vi "UpdateStatusChannels.vi"(8 "error in (no error)":errorcluster, 9 "success?":bool, 10 "Data":u8[](array[numeric]), 11 "StatusFIFO":refnum<k33>) -> (0 "error out":errorcluster)   [LabVIEW 2015, in "Diagnostics Addon Engine.lvlib"]
uses:
  Diagnostics Addon Engine.lvlib
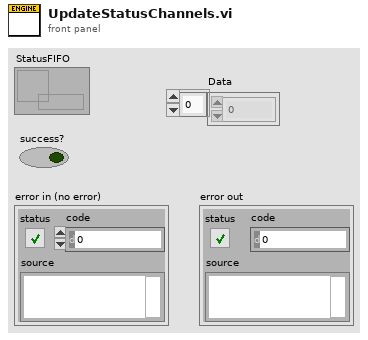
[diagram p1: front panel]
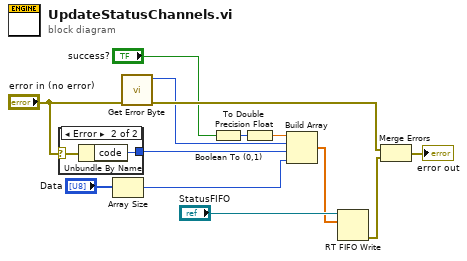
[diagram p0: block diagram]
diagram:
  n1 = case shown="Error" "error in (no error)" {
    selector: "error in (no error)" -> [_ w15]
    tunnel: [_ w14] -> w3
    frame No Error {
    }
    frame Error {
      n2 = Unbundle By Name(w15) -> ("code"=w14:i32)
    }
  }
  n3 = Array Size(array="Data") -> (size(s)=w2:i32)
  n4 = call "Get Error Byte.vi"("error"="error in (no error)") -> ("error  out"=w13:errorcluster, "Error Byte"=w4:u8)  [unwired: 9 in]
  n5 = Boolean To (0,1)(Boolean="success?") -> (0, 1=w6:i16)
  n6 = To Double Precision Float(number=w6) -> (double precision float=w7:dbl)
  n7 = Build Array(w7, w4, w3, w2) -> (w1:dbl[])
  n8 = RT FIFO Write(0:"StatusFIFO", 1:w1) -> (11:w10:errorcluster)  [unwired: 3 in, 3 out]
  n9 = Merge Errors(w13, w10) -> (→"error out":errorcluster)
